vi "Write FPGA_Ref.vi"(8 "error in":errorcluster, 10 "FPGA VI Reference Out":T1, 11 "Combined PAS in":refnum<class "cPAS.lvclass">) -> (0 "error out":errorcluster, 3 "Combined PAS out":refnum<class "cPAS.lvclass">)   [LabVIEW 2015, in "cPAS.lvclass"]
uses:
  cPAS.lvclass
  Interface/fpga_ctl.ctl
  cPAS.lvclass/cPAS.ctl
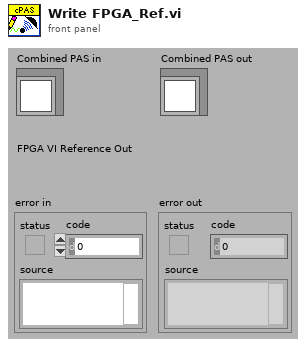
[diagram p1: front panel]
types:
  T1 = typedef "fpga_ctl.ctl" = refnum<k20>
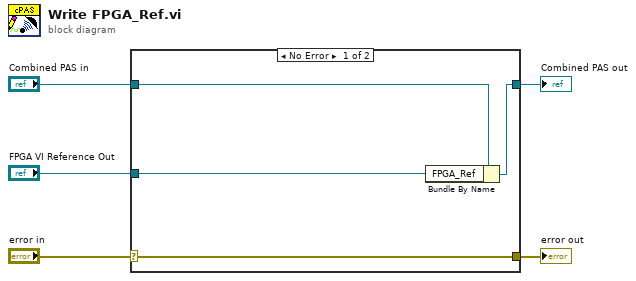
[diagram p0: block diagram]
diagram:
  n1 = case shown="No Error" "error in" {
    selector: "error in" -> [w9 w10]
    tunnel: [w9 w10] -> w4
    tunnel: [w7 w11] -> w2
    tunnel: "Combined PAS in" -> [w8 w11]
    tunnel: "FPGA VI Reference Out" -> [w6 _]
    frame No Error {
      n2 = Bundle By Name(cluster=w8, "FPGA_Ref"=w6) -> (w7:refnum<class "cPAS.lvclass">)
    }
    frame Error {
    }
  }
  "error out" <- w4
  "Combined PAS out" <- w2
